vi "Convert Seconds To Milliseconds.vi"(11 "Seconds":dbl) -> (3 "Milliseconds":dbl)   [LabVIEW 2022 SP3, in "Utility.lvlib"]
uses:
  Utility.lvlib
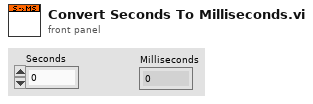
[diagram p1: front panel]
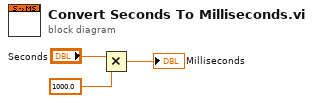
[diagram p0: block diagram]
diagram:
  n1 = Multiply(x="Seconds", y=1000.0) -> (x*y=→"Milliseconds":dbl)
